vi "CalculateRunningAverage.vi"(7 "WeightOfNewFrequency":dbl=0.1 format="%#_13g", 11 "ToneClustIn":T1={"Shift_"=0.0, "Peak_ToFPGA"=0.0, "MaxValue"=0.0, "MaxIndex"=0, "Tone"={"PkLocTrak"=0.0, "PkLocDisp"=0.0, "df_"=0.0, "ZoomPwr"=[], "Phase"=0.0, "PhaseOld"=0.0, "AboveThresh?"=FALSE, "MaxI"=0.0, "MaxQ"=0.0, "median"=0.0, "ISpect"=[], "QSpect"=[], "DeltaPhase"=0.0}, "TimeDomainI"=[], "TimeDomainQ"=array[12500 elements], "PwrSpectrum"=[], "RunningAvgFreq"=0.0, "ISpectPos"=[], "ISpectNeg"=[], "QSpectPos"=[], "QSpectNeg"=[], "10Hz_PwrSpectr"=[], "SNR"=0.0, "AliasWarn"=FALSE, "10Hz_Peak"=[], "ISpect+-"=[], "QSpect+-"=[], "TimeStamp"=timestamp(0 s since 1904-01-01), "I_Index"=array[12500 elements], "Q_Index"=array[12500 elements], "10MHz"=FALSE} {"Tone"."median" format="%0.2f"; "Tone"."MaxQ" format="%0.2f"}) -> (0 "RunningAvgFreq":dbl, 2 "NewRunningAverage":dbl, 3 "ToneClustOut":T1 {"Tone"."median" format="%0.2f"; "Tone"."MaxQ" format="%0.2f"}, 4 "Tone.PeakLoc":dbl)   [LabVIEW 2018]
uses:
  Controls/Clusts/ChannelToneData.ctl
  Controls/ToneInfoClust.ctl
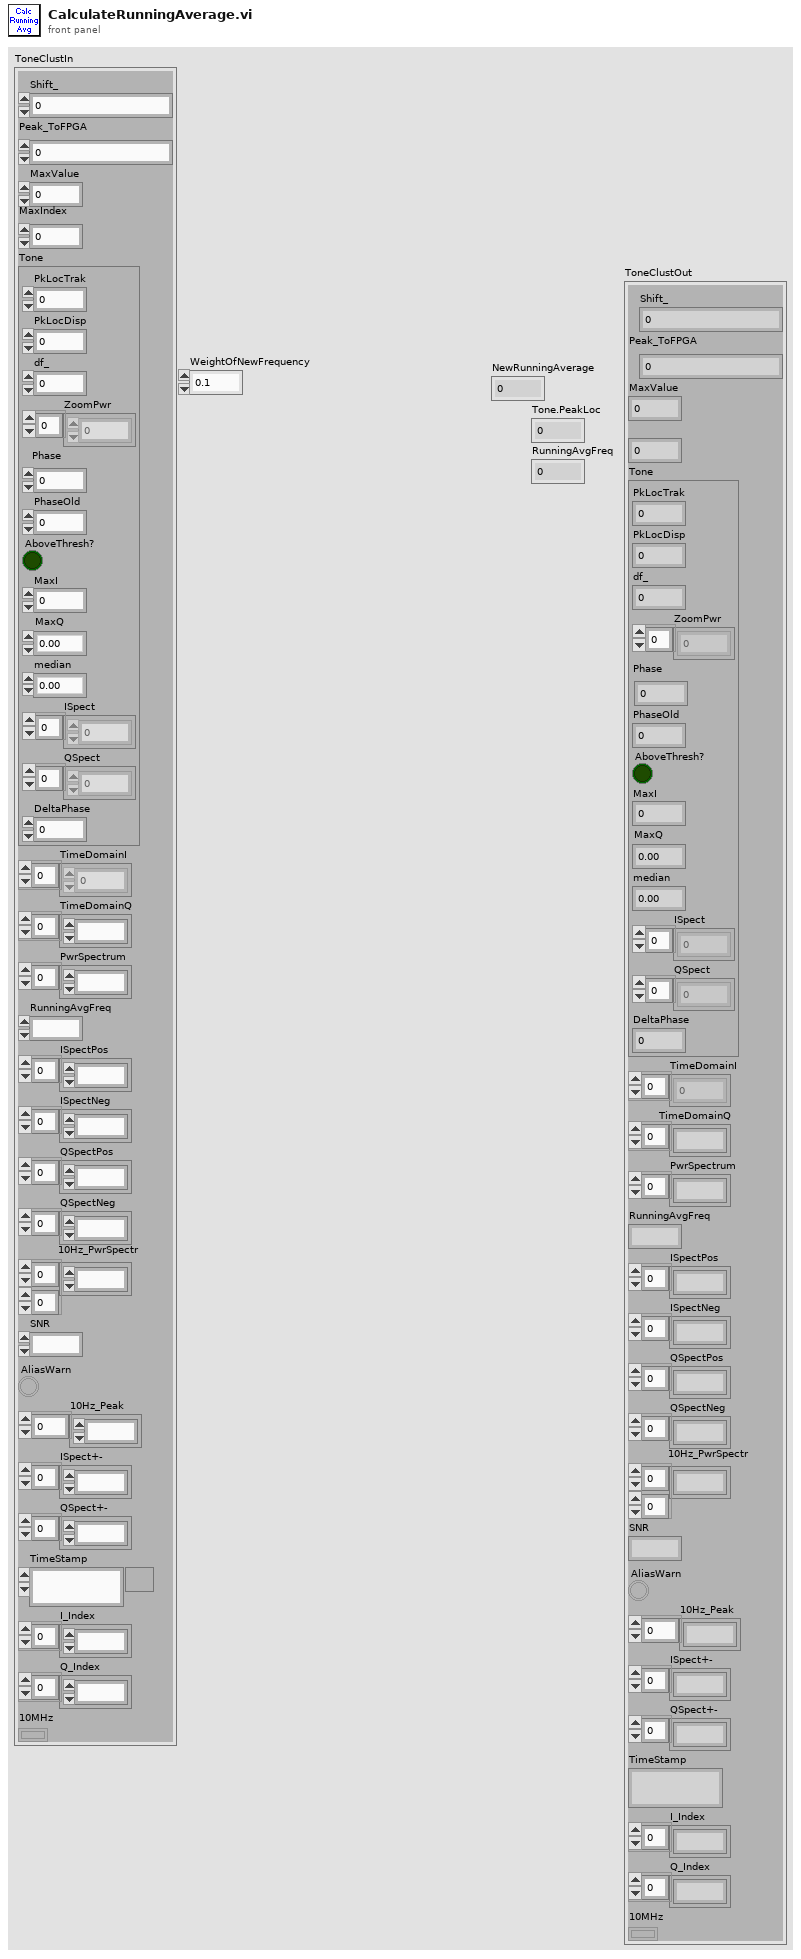
[diagram p1: front panel]
types:
  T1 = typedef "ChannelToneData.ctl" = cluster{"Shift_":dbl, "Peak_ToFPGA":dbl, "MaxValue":dbl, "MaxIndex":i32, "Tone":T2, "TimeDomainI":ext[], "TimeDomainQ":ext[], "PwrSpectrum":dbl[], "RunningAvgFreq":dbl, "ISpectPos":dbl[], "ISpectNeg":dbl[], "QSpectPos":dbl[], "QSpectNeg":dbl[], "10Hz_PwrSpectr":dbl[][], "SNR":dbl, "AliasWarn":bool, "10Hz_Peak":dbl[], "ISpect+-":dbl[], "QSpect+-":dbl[], "TimeStamp":timestamp, "I_Index":ext[], "Q_Index":ext[], "10MHz":bool}
  T2 = typedef "ToneInfoClust.ctl" = cluster{"PkLocTrak":dbl, "PkLocDisp":dbl, "df_":dbl, "ZoomPwr":dbl[], "Phase":dbl, "PhaseOld":dbl, "AboveThresh?":bool, "MaxI":dbl, "MaxQ":dbl, "median":dbl, "ISpect":dbl[], "QSpect":dbl[], "DeltaPhase":dbl}
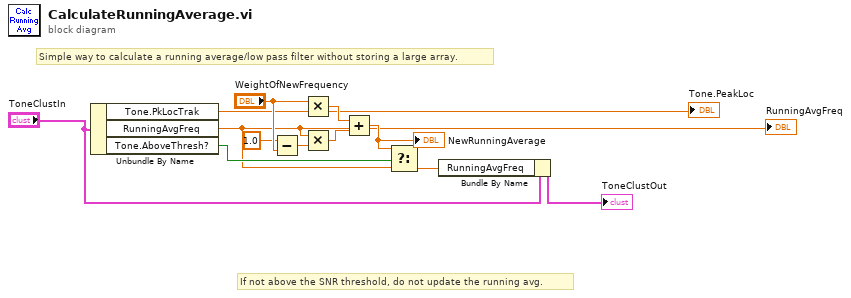
[diagram p0: block diagram]
diagram:
  # "If not above the SNR threshold, do not update the running avg."
  # "Simple way to calculate a running average/low pass filter without storing a large array."
  n1 = Unbundle By Name("ToneClustIn") -> ("Tone.PkLocTrak"=w2:dbl, "RunningAvgFreq"=w1:dbl, "Tone.AboveThresh?"=w3:bool)
  "Tone.PeakLoc" <- w2
  "RunningAvgFreq" <- w1
  n2 = Subtract(x=1.0 ("y"), y="WeightOfNewFrequency") -> (x-y=w8:dbl)
  n3 = Multiply(x="WeightOfNewFrequency", y=w2) -> (x*y=w12:dbl)
  n4 = Multiply(x=w1, y=w8) -> (x*y=w11:dbl)
  n5 = Add(x=w12, y=w11) -> (x+y=w4:dbl)
  "NewRunningAverage" <- w4
  n6 = Select(t=w4, s=w3, f=w1) -> (s? t:f=w5:dbl)
  n7 = Bundle By Name(cluster="ToneClustIn", "RunningAvgFreq"=w5) -> (→"ToneClustOut":T1)
